vi "HOST.vi"() -> ()   [LabVIEW 2013]
uses:
  <instrlib>/niDCPower/nidcpower.llb/niDCPower Measurement Type.ctl
panel:
  in  "GEN_ON":bool
  in  "Контроль U_IN":bool
  in  "Контроль тока утечки":bool
  in  "V_OUT_ON":bool
  in  "Power":refnum<k15>="Dev2" caption="instrument handle"
  in  "LOGS":path=path "C:/VPL/LabView_PRJ/НИИ ТВ/LOGS"
  out "Номер образца":string="0"
  out "V_IN_cur":dbl=1.4842482521625679e-05 caption="measurement" format="%_6g"
  out "V_OUT_cur":dbl=0.00013018728653541934 caption="measurement" format="%_6g"
  in  "V_IN_ON":bool
  out "V_IN_char":dbl(graph)=1.4842482521625679e-05
  out "V_OUT_char":dbl(graph)=0.00013018728653541934
  in  "Стоп":bool
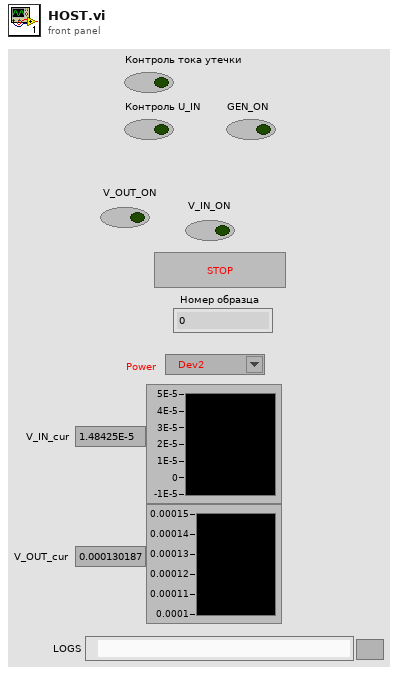
[diagram p1: front panel]
types:
  T1 = enum16{"open", "replace", "create", "open or create", "replace or create", "replace or create with confirmation"}
  T2 = typedef "niDCPower Measurement Type.ctl" = i32
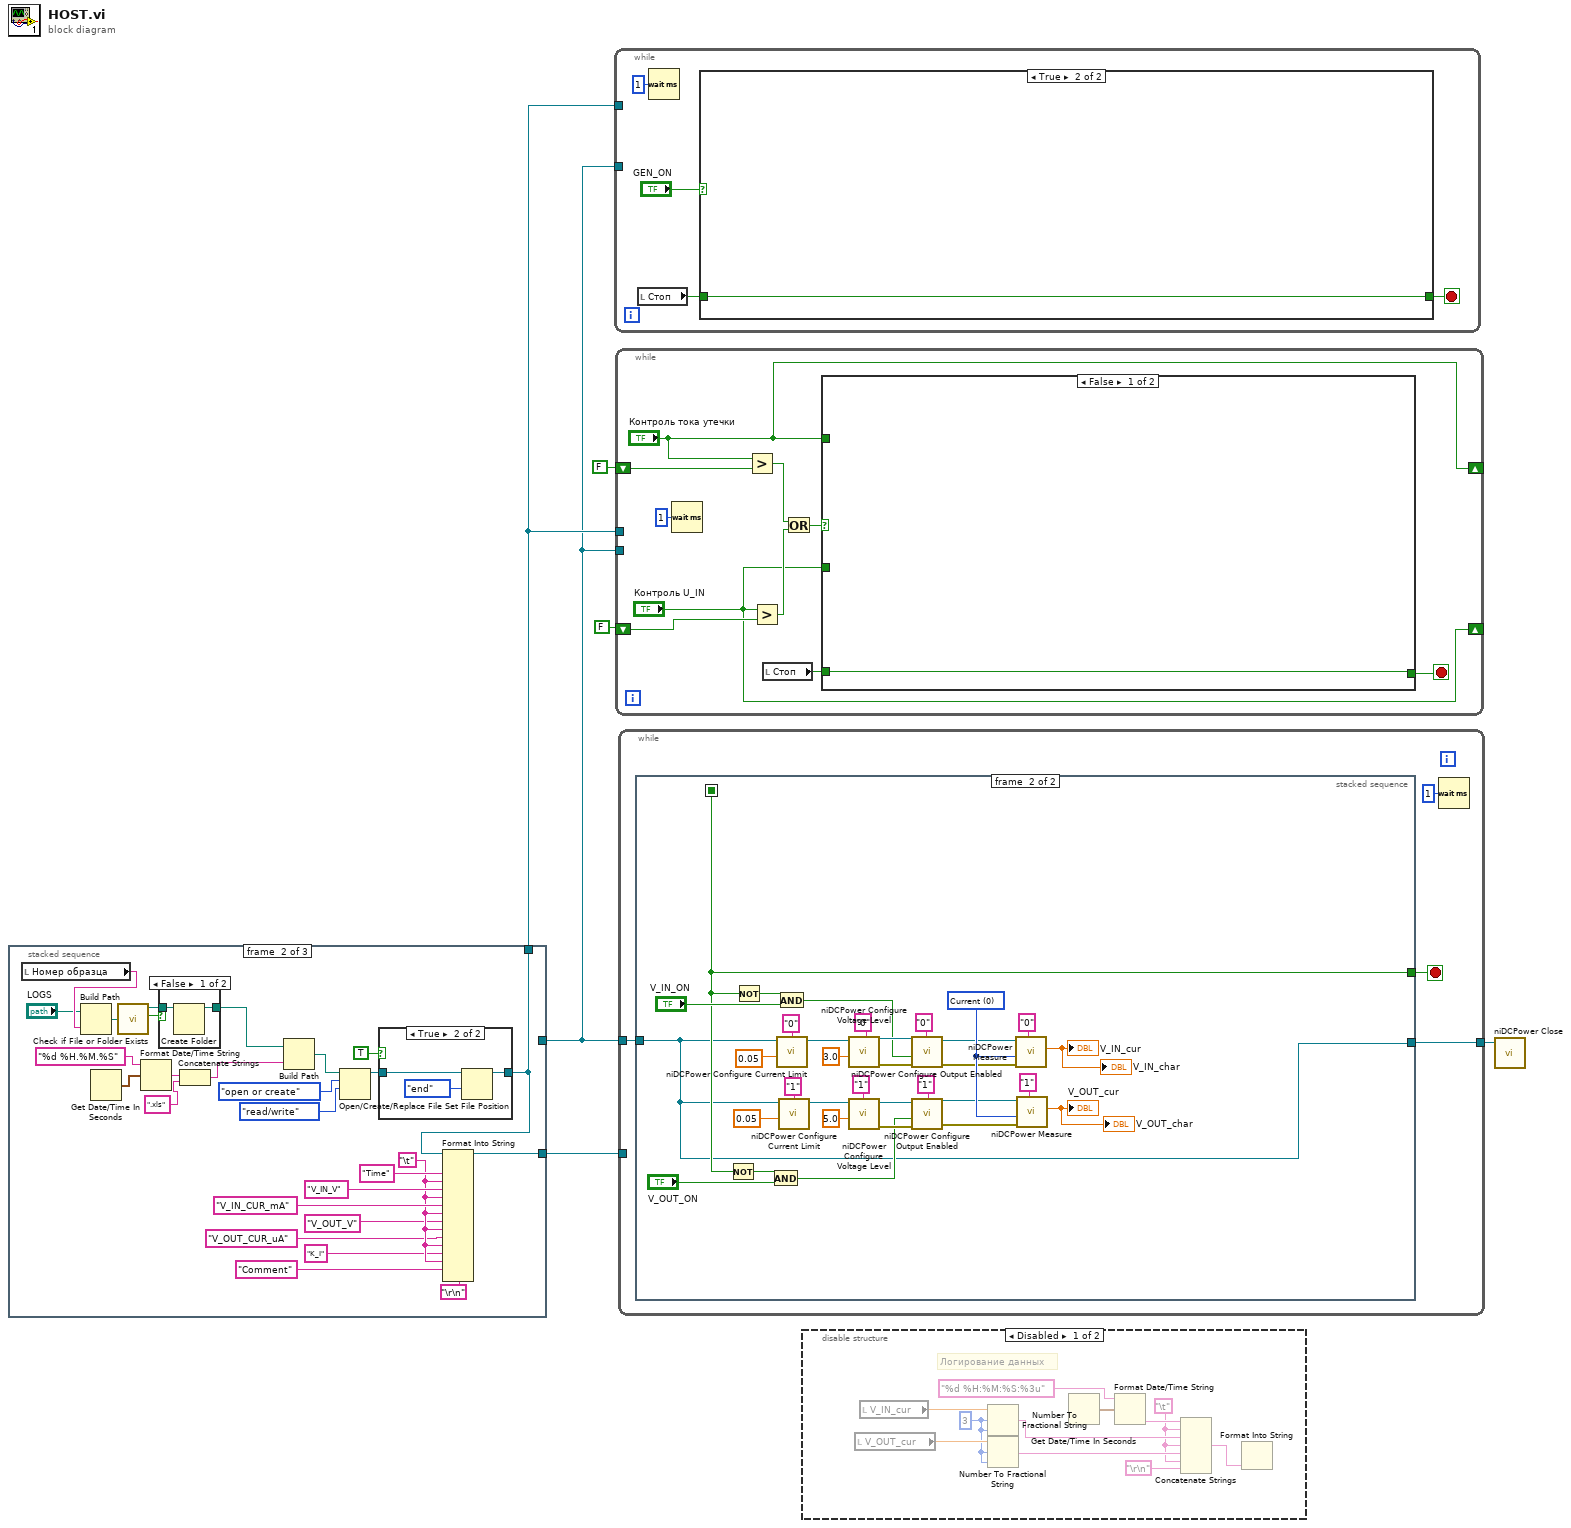
[diagram p0: block diagram]
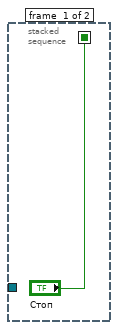
[diagram p5: hidden frame]
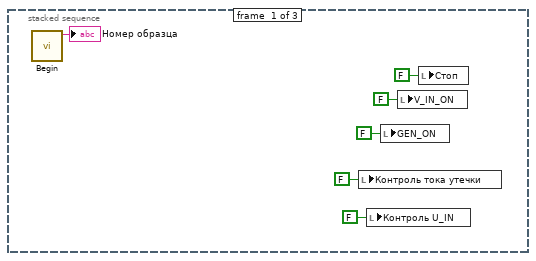
[diagram p6: hidden frame]
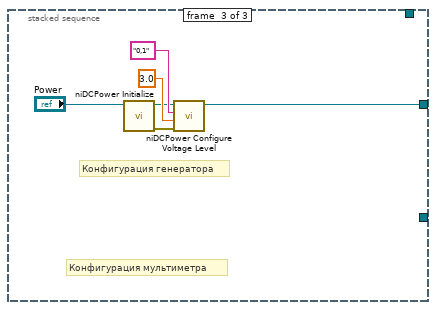
[diagram p9: hidden frame]
diagram:
  n1 = stacked-sequence {
    tunnel: [_ _ w47] -> w1
    tunnel: [_ w20 _] -> w6
    tunnel: [_ w13 _] -> w2
    frame #0 {
      n2 = call "Begin.vi"() -> ("Номер образца 2"=→"Номер образца":string)  [unwired: 11 in]
      n3 = local write "Контроль тока утечки"(FALSE ("Контроль тока утечки")) -> ()
      n4 = local write "Контроль U_IN"(FALSE ("Контроль U_IN")) -> ()
      n5 = local write "GEN_ON"(FALSE ("GEN_ON")) -> ()
      n6 = local write "V_IN_ON"(FALSE ("Питание")) -> ()
      n7 = local write "Стоп"(FALSE ("Стоп")) -> ()
    }
    frame #1 {
      w19 = "\t"
      n8 = local read "Номер образца"() -> (w39:string)
      n9 = Build Path(base path="LOGS", name or relative path=w39) -> (appended path=w36:path)
      n10 = Get Date/Time In Seconds() -> (seconds since 1Jan1904=w33:timestamp)
      n11 = call <vilib>:"Check if File or Folder Exists.vi"("path"=w36) -> ("file or folder exists?"=w37:bool, "dup path"=w38:path)  [unwired: 8 in, 1 out]
      n12 = Format Date/Time String(time format string (%c)="%d %H.%M.%S", seconds (now)=w33) -> (date/time string=w31:string)  [unwired: 1 in]
      n13 = case shown="False" w37 {
        tunnel: w38 -> [w45 w46]
        tunnel: [w44 w46] -> w29
        frame False {
          n14 = Create Folder(path (use dialog)=w45) -> (created path=w44:path)  [unwired: 2 in, 2 out]
        }
        frame True {
        }
      }
      n15 = Concatenate Strings(w31, ".xls" ("string")) -> (w30:string)
      n16 = Build Path(base path=w29, name or relative path=w30) -> (appended path=w32:path)
      n17 = Open/Create/Replace File(file path (use dialog)=w32, operation (0:open)=T1."open or create", access (0:read/write)=enum16{"read/write", "read-only", "write-only"}."read/write") -> (refnum out=w34:refnum<file>)  [unwired: 3 in, 2 out]
      n18 = case shown="True" TRUE {
        tunnel: w34 -> [w40 w43]
        tunnel: [w40 w41] -> w13
        frame False {
        }
        frame True {
          n19 = Set File Position(refnum=w43, from (0:start)=enum16{"start", "end", "current"}."end") -> (refnum out=w41:refnum<file>)  [unwired: 2 in, 1 out]
        }
      }
      n20 = Format Into String(initial string=w13, "Time" ("input 1"), w19, "V_IN_V", w19, "V_IN_CUR_mA", w19, "V_OUT_V", w19, "V_OUT_CUR_uA", w19, "K_I", w19, "Comment", "\r\n") -> (resulting string=w20:refnum<file>)  [unwired: 2 in, 1 out]
    }
    frame #2 {
      # "Конфигурация мультиметра"
      # "Конфигурация генератора"
      n21 = call <instrlib>:"niDCPower Initialize.vi"("resource name"="Power") -> ("error out"=w49:errorcluster, "instrument handle out"=w48:refnum<k15>)  [unwired: 3 in, 6 out]
      n22 = call <instrlib>:"niDCPower Configure Voltage Level.vi"("error in (no error)"=w49, "voltage level"=3.0, "channel name"="0,1", "instrument handle"=w48) -> ("instrument handle out"=w47:refnum<k15>)  [unwired: 6 in, 1 out]
    }
  }
  n23 = while {
    tunnel: w2 -> [_]
    tunnel: w1 -> [_]
    stop <- w55 stop-if-true
    n24 = local read "Стоп"() -> (w54:bool)
    n25 = Wait (ms)(milliseconds to wait=u32 1) -> ()  [unwired: 1 out]
    n26 = case shown="True" "GEN_ON" {
      tunnel: [w57 w58] -> w55
      tunnel: w54 -> [w57 w58]
      frame False {
      }
      frame True {
      }
    }
  }
  n27 = while {
    shift-right: ["Контроль тока утечки"] -> _
    shift-left: FALSE -> [w66]
    shift-right: ["Контроль U_IN"] -> _
    shift-left: FALSE -> [w65]
    tunnel: w2 -> [_]
    tunnel: w1 -> [_]
    stop <- w60 stop-if-true
    n28 = Wait (ms)(milliseconds to wait=u32 1) -> ()  [unwired: 1 out]
    n29 = Greater?(x="Контроль тока утечки", y=w66) -> (0:w64:bool)
    n30 = Greater?(x="Контроль U_IN", y=w65) -> (0:w63:bool)
    n31 = local read "Стоп"() -> (w59:bool)
    n32 = Or(x=w64, y=w63) -> (x .or. y?=w67:bool)
    n33 = case shown="False" w67 {
      tunnel: "Контроль тока утечки" -> [_ _]
      tunnel: "Контроль U_IN" -> [_ _]
      tunnel: [w69 w70] -> w60
      tunnel: w59 -> [w69 w70]
      frame False {
      }
      frame True {
      }
    }
  }
  n34 = while {
    tunnel: [w72] -> w5
    tunnel: w1 -> [w71]
    tunnel: w6 -> [_]
    stop <- w73 stop-if-true
    n35 = stacked-sequence {
      seq-local: ["Стоп" _] -> [_ w88]
      tunnel: [_ w80] -> w72
      tunnel: [_ w88] -> w73
      tunnel: w71 -> [_ w80]
      frame #0 {
      }
      frame #1 {
        w83 = T2 0 items=["Current", "Voltage"] ("measurement type")
        n36 = Not(x=w88) -> (.not. x?=w89:bool)
        n37 = Not(x=w88) -> (.not. x?=w96:bool)
        n38 = And(x=w89, y="V_OUT_ON") -> (x .and. y?=w86:bool)
        n39 = And(x=w96, y="V_IN_ON") -> (x .and. y?=w94:bool)
        n40 = call <instrlib>:"niDCPower Configure Current Limit.vi"("current limit"=0.05 ("V_OUT_curlim"), "channel name"="0", "instrument handle"=w80) -> ("instrument handle out"=w107:refnum<k15>)  [unwired: 7 in, 1 out]
        n41 = call <instrlib>:"niDCPower Configure Current Limit.vi"("current limit"=0.05 ("V_OUT_curlim"), "channel name"="1", "instrument handle"=w80) -> ("instrument handle out"=w108:refnum<k15>)  [unwired: 7 in, 1 out]
        n42 = call <instrlib>:"niDCPower Configure Voltage Level.vi"("voltage level"=3.0, "channel name"="0", "instrument handle"=w107) -> ("error out"=w101:errorcluster, "instrument handle out"=w104:refnum<k15>)  [unwired: 7 in]
        n43 = call <instrlib>:"niDCPower Configure Voltage Level.vi"("voltage level"=5.0, "channel name"="1", "instrument handle"=w108) -> ("error out"=w102:errorcluster, "instrument handle out"=w103:refnum<k15>)  [unwired: 7 in]
        n44 = call <instrlib>:"niDCPower Configure Output Enabled.vi"("error in (no error)"=w101, "output enabled"=w94, "channel name"="0", "instrument handle"=w104) -> ("error out"=w76:errorcluster, "instrument handle out"=w79:refnum<k15>)  [unwired: 6 in]
        n45 = call <instrlib>:"niDCPower Configure Output Enabled.vi"("error in (no error)"=w102, "output enabled"=w86, "channel name"="1", "instrument handle"=w103) -> ("error out"=w77:errorcluster, "instrument handle out"=w78:refnum<k15>)  [unwired: 6 in]
        n46 = call <instrlib>:"niDCPower Measure.vi"("error in (no error)"=w76, "measurement type"=w83, "channel name"="0", "instrument handle"=w79) -> ("measurement"=→"V_IN_cur" →"V_IN_char":dbl)  [unwired: 5 in, 2 out]
        n47 = call <instrlib>:"niDCPower Measure.vi"("error in (no error)"=w77, "measurement type"=w83, "channel name"="1", "instrument handle"=w78) -> ("measurement"=→"V_OUT_cur" →"V_OUT_char":dbl)  [unwired: 5 in, 2 out]
      }
    }
    n48 = Wait (ms)(milliseconds to wait=u32 1) -> ()  [unwired: 1 out]
  }
  n49 = disable-structure shown="Disabled" {
    frame Disabled {
      w111 = i16 3 ("width (-)")
      w110 = "\t"
      # "Логирование данных"
      n50 = local read "V_OUT_cur"() -> (w119:dbl)
      n51 = local read "V_IN_cur"() -> (w118:dbl)
      n52 = Number To Fractional String(number=w118, width (-)=w111, precision (6)=w111) -> (F-format string=w116:string)  [unwired: 1 in]
      n53 = Number To Fractional String(number=w119, width (-)=w111, precision (6)=w111) -> (F-format string=w117:string)  [unwired: 1 in]
      n54 = Get Date/Time In Seconds() -> (seconds since 1Jan1904=w113:timestamp)
      n55 = Format Date/Time String(time format string (%c)="%d %H:%M:%S:%3u", seconds (now)=w113) -> (date/time string=w115:string)  [unwired: 1 in]
      n56 = Concatenate Strings(w115, w110, w116, w110, w117, w110, "\r\n") -> (w114:string)
      n57 = Format Into String(w114) -> ()  [unwired: 3 in, 2 out]
    }
    frame Enabled {
    }
  }
  n58 = call <instrlib>:"niDCPower Close.vi"("instrument handle"=w5) -> ()  [unwired: 10 in, 1 out]
